vi "uSubscription Destruct.vi"(8 "error in (no error)":errorcluster, 11 "uSubscription in":refnum<class "uSubscription.lvclass">) -> (0 "error out":errorcluster)   [LabVIEW 2023, in "uFramework.lvlib" / "uSubscription.lvclass"]
uses:
  uSubscription.lvclass
  uSubscription.lvclass/uSubscription.ctl
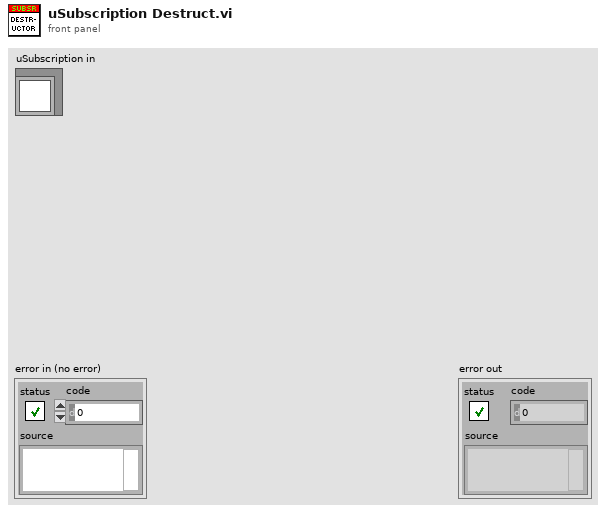
[diagram p1: front panel]
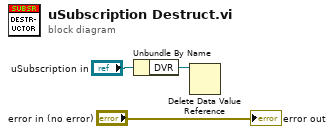
[diagram p0: block diagram]
diagram:
  n1 = Unbundle By Name("uSubscription in") -> ("DVR"=w1:refnum<data-value>)
  n2 = Delete Data Value Reference(data value reference=w1) -> ()  [unwired: 1 in, 2 out]
  "error out" <- "error in (no error)"
